vi "XYZStage-Z-axis safety interlock.vi"(3 "Z":sgl) -> (1 "Z":sgl)   [LabVIEW 2013]
uses:
  User Interface/Windows/Position control window/Globals/Pos ctrl window globals.vi
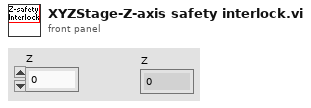
[diagram p1: front panel]
types:
  T1 = typedef "Imaging Protocols enum.ctl" = enum16{"AOL Z-Stack", "Motor Z Stack", "Functional Acquisition", "Single Plane Acquisition", "Volume Acquisition", "Live Imaging", "Live Plane Imaging", "Live Volume Imaging"}
  T2 = cluster{"Caption-Right button":string, "Caption-Left button":string, "Message to display":string, "Delay before close":u32, "Window Colour":u32, "Cancel button disabled?":enum8{"Enabled", "Disabled", "Disabled and Grayed Out"}}
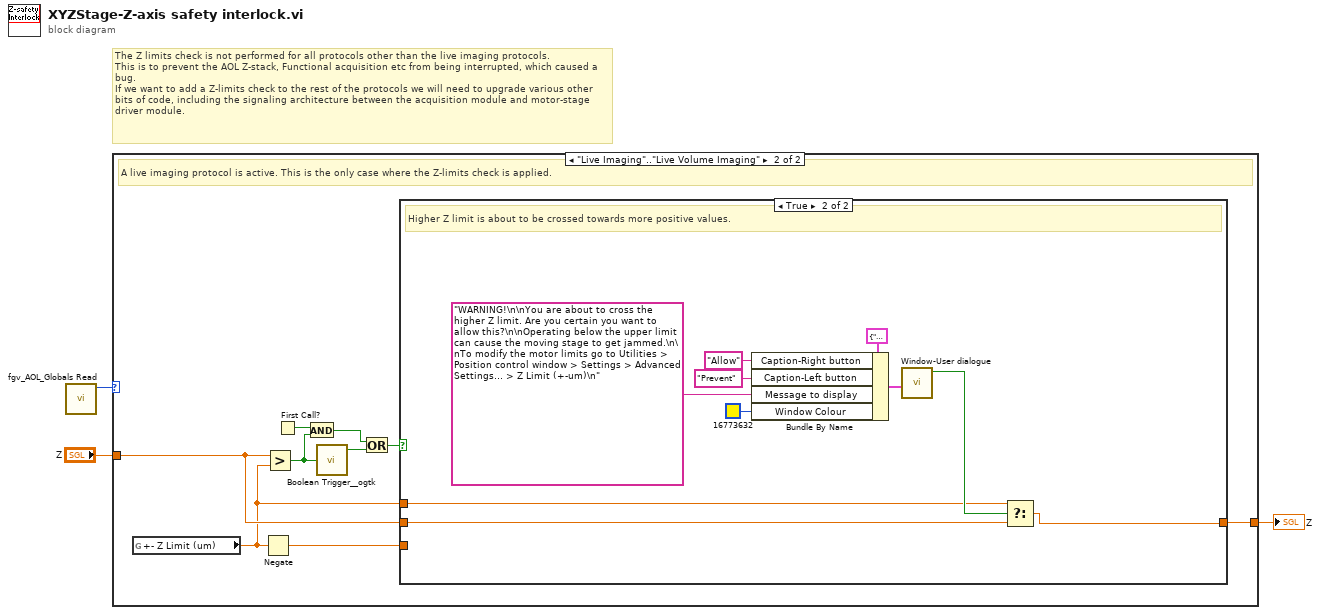
[diagram p0: block diagram]
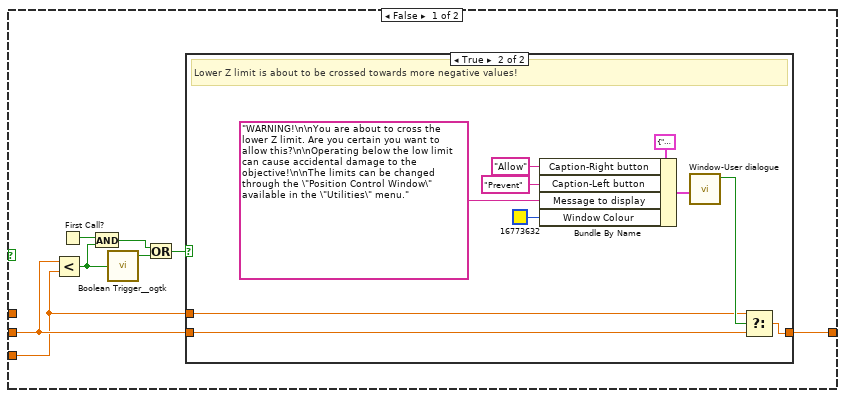
[diagram p3: hidden frame]
diagram:
  # "The Z limits check is not performed for all protocols other than the live imaging protocols.\nThis is to prevent the AOL Z-stack, Functional acquisition etc from being interrupted, which caused a bug.\nIf we want to add a Z-limits check to the rest of the protocols we will need to upgrade various other bits of code, including the signaling architecture between the acquisition module and motor-stage driver module."
  n1 = call "fgv_AOL_Globals Read.vi"() -> ("Imaging Protocol"=w1:T1)  [unwired: 9 in, 2 out]
  n2 = case shown="\"Live Imaging\"..\"Live Volume Imaging\"" w1 {
    tunnel: [w4 w13] -> w3
    tunnel: "Z" -> [w4 w12]
    frame Default {
      # "Do nothing. No Z-limits check for all protocols other than the live imaging protocols."
    }
    frame "Live Imaging".."Live Volume Imaging" {
      # "A live imaging protocol is active. This is the only case where the Z-limits check is applied."
      n3 = global read "Pos ctrl window globals.vi" "+- Z Limit (um)"() -> (w11:sgl)
      n4 = Negate(x=w11) -> (-x=w10:sgl)
      n5 = Greater?(x=w12, y=w11) -> (0:w8:bool)
      n6 = First Call?() -> (First Call?: T/F=w9:bool)
      n7 = And(x=w9, y=w8) -> (x .and. y?=w6:bool)
      n8 = call "Boolean Trigger__ogtk.vi"("Boolean Input"=w8) -> ("Rising Edge"=w7:bool)  [unwired: 1 in, 1 out]
      n9 = Or(x=w6, y=w7) -> (x .or. y?=w5:bool)
      n10 = case shown="True" w5 {
        tunnel: w12 -> [w20 w42]
        tunnel: [w21 w41] -> w13
        tunnel: w11 -> [_ w39]
        tunnel: w10 -> [w19 _]
        frame False {
          n11 = Less?(x=w20, y=w19) -> (x < y?=w18:bool)
          n12 = First Call?() -> (First Call?: T/F=w17:bool)
          n13 = And(x=w17, y=w18) -> (x .and. y?=w14:bool)
          n14 = call "Boolean Trigger__ogtk.vi"("Boolean Input"=w18) -> ("Rising Edge"=w16:bool)  [unwired: 1 in, 1 out]
          n15 = Or(x=w14, y=w16) -> (x .or. y?=w15:bool)
          n16 = case shown="True" w15 {
            tunnel: w20 -> [w22 w32]
            tunnel: [w22 w31] -> w21
            tunnel: w19 -> [_ w29]
            frame False {
            }
            frame True {
              # "Lower Z limit is about to be crossed towards more negative values!"
              n17 = Bundle By Name(cluster=T2 {"Caption-Right button"="", "Caption-Left button"="", "Message to display"="", "Delay before close"=0, "Window Colour"=16448250, "Cancel button disabled?"=enum."Enabled"} ("Input cluster"), "Caption-Right button"="Allow", "Caption-Left button"="Prevent", "Message to display"="WARNING!\n\nYou are about to cross the lower Z limit. Are you certain you want to allow this?\n\nOperating below the low limit can cause accidental damage to the objective!\n\nThe limits can be changed through the \"Position Control Window\" available in the \"Utilities\" menu." ("Message string"), "Window Colour"=u32 16773632) -> (w24:T2)
              n18 = call "Window-User dialogue.vi"("Input cluster"=w24) -> ("Left Button (Cancel)"=w30:bool)  [unwired: 10 in]
              n19 = Select(t=w29, s=w30, f=w32) -> (s? t:f=w31:sgl)
            }
          }
        }
        frame True {
          # "Higher Z limit is about to be crossed towards more positive values."
          n20 = Bundle By Name(cluster=T2 {"Caption-Right button"="", "Caption-Left button"="", "Message to display"="", "Delay before close"=0, "Window Colour"=16448250, "Cancel button disabled?"=enum."Enabled"} ("Input cluster"), "Caption-Right button"="Allow", "Caption-Left button"="Prevent", "Message to display"="WARNING!\n\nYou are about to cross the higher Z limit. Are you certain you want to allow this?\n\nOperating below the upper limit can cause the moving stage to get jammed.\n\nTo modify the motor limits go to Utilities > Position control window > Settings > Advanced Settings… > Z Limit (+-um)\n" ("Message string"), "Window Colour"=u32 16773632) -> (w34:T2)
          n21 = call "Window-User dialogue.vi"("Input cluster"=w34) -> ("Left Button (Cancel)"=w40:bool)  [unwired: 10 in]
          n22 = Select(t=w39, s=w40, f=w42) -> (s? t:f=w41:sgl)
        }
      }
    }
  }
  "Z" <- w3
